vi "FPGAcode2_redo.vi"() -> ()   [LabVIEW 2015]
uses:
  IO_Cluster.ctl
  Limits_In.ctl
  <vilib>/Platform/TimedLoop/XDataNode/timing_clust.ctl
  <vilib>/Platform/TimedLoop/XDataNode/nitl_modes.ctl
  <vilib>/Platform/TimedLoop/XDataNode/wakeup.ctl
  <vilib>/rvi/Emulation/niFpgaGetClockAttributes.vi
  <vilib>/rvi/Emulation/niFpgaSctlEmulationGetInTimedLoop.vi
  <vilib>/rvi/Emulation/niFpgaEmulationReportErrorSimple.vi
  <vilib>/rvi/Emulation/niFpgaProcessEmulError.vi
  <vilib>/rvi/eio/common/nirviEmuTemplateMethod_errors.vi
  <vilib>/rvi/Emulation/niFpgaCriticalErrorInLSC.vi
  <vilib>/eio/EIONode/EIONode.xnode
  <vilib>/Platform/TimedLoop/XDataNode/XDataNode.xnode
  <vilib>/Platform/TimedLoop/XDataNode/XDNodeRunTimeDep.lvlib
panel:
  out "Delay":bool
  out "Plates":bool
  out "Offset Average":i16
  out "Boxcar Average":i16
  in  "Filter Thresholds":T1
  in  "Limits In":T2
  out "Detector 3 Correlations":T1
  out "Detector 1 Correlations":T1
  out "Del Armed":bool[](array[boolean])
  out "Armed":bool[](array[boolean])
  out "Delay Array":bool[](array[boolean])
  out "Plates Array":bool[](array[boolean])
  in  "Reset One Shot":bool
  in  "One Shot":bool
  in  "Mult1":fxp<+,16,7>
  out "IO Module\\AI 0":i16
  out "IO Module\\AI 1":i16
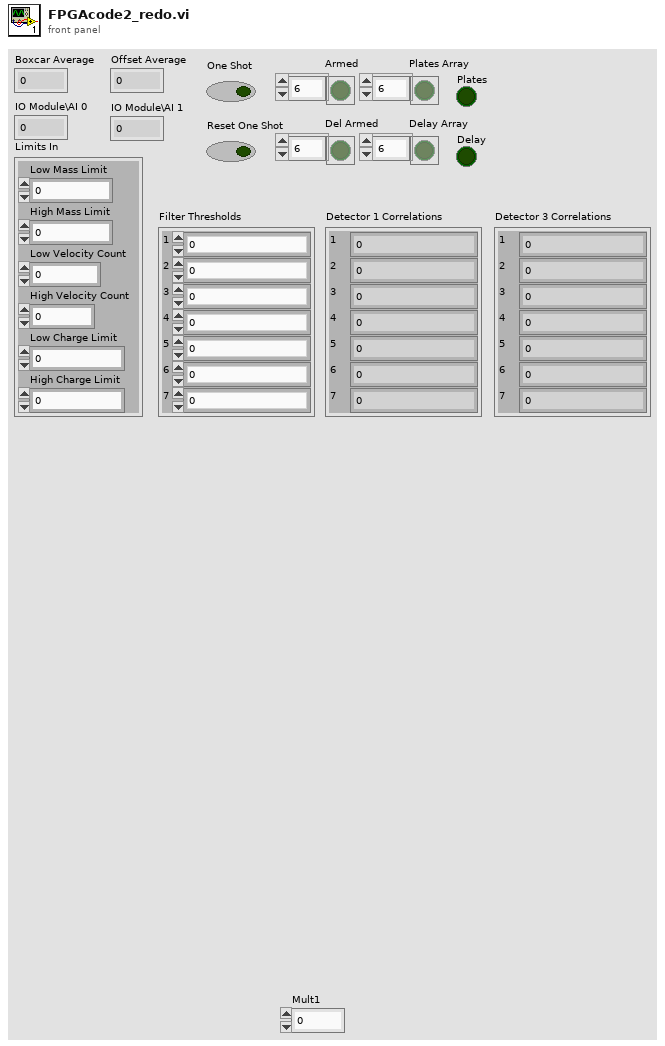
[diagram p1: front panel]
types:
  T1 = typedef "IO_Cluster.ctl" = cluster{"1":i16, "2":i16, "3":i16, "4":i16, "5":i16, "6":i16, "7":i16}
  T2 = typedef "Limits_In.ctl" = cluster{"Low Mass Limit":i64, "High Mass Limit":i64, "Low Velocity Count":i32, "High Velocity Count":i32, "Low Charge Limit":i16, "High Charge Limit":i16}
  T3 = typedef "XDNodeRunTimeDep.lvlib/timing_clust.ctl" = cluster{"Expected End [f-1]":u64, "Actual End [f-1]":u64, "Finished Late? [f-1]":bool, "Expected End [i-1]":u64, "Actual End [i-1]":u64, "Finished Late? [i-1]":bool, "Expected Start [i]":u64, "Actual Start [i]":u64, "Expected Start [f]":u64, "Actual Start [f]":u64, "Source Name":string, "Structure Name":string, "Period":i64, "Deadline":i64, "Offset":i64, "Start":i64, "Priority":i32, "Timeout":i32, "Mode":T4, "Wakeup Reason":T5, "Error":errorcluster, "Source Type":string, "Secondary Source Type":string, "Global End Time":u64, "Global Start Time":u64, "Frame Duration":u64, "Iteration Duration":u64, "Assigned CPU":i32, "I/O Scan Engine Mode":u32}
  T4 = typedef "XDNodeRunTimeDep.lvlib/nitl_modes.ctl" = enum32{"No Change", "Process missed periods, maintain original phase", "Discard missed periods, maintain original phase", "Process missed periods, ignore original phase", "Discard missed periods, ignore original phase"}
  T5 = typedef "XDNodeRunTimeDep.lvlib/wakeup.ctl" = enum32{"Normal", "Aborted", "Asynchronous wakeup", "Timing source error", "Timed loop error", "Timeout"}
  T6 = cluster{"High Charge Limit":i16, "Low Charge Limit":i16, "Time Out Limit":i32, "High Velocity Count":i32, "Low Velocity Count":i32, "Sampling Rate":fxp<+,30,25>, "High Mass Limit":i64, "Low Mass Limit":i64}
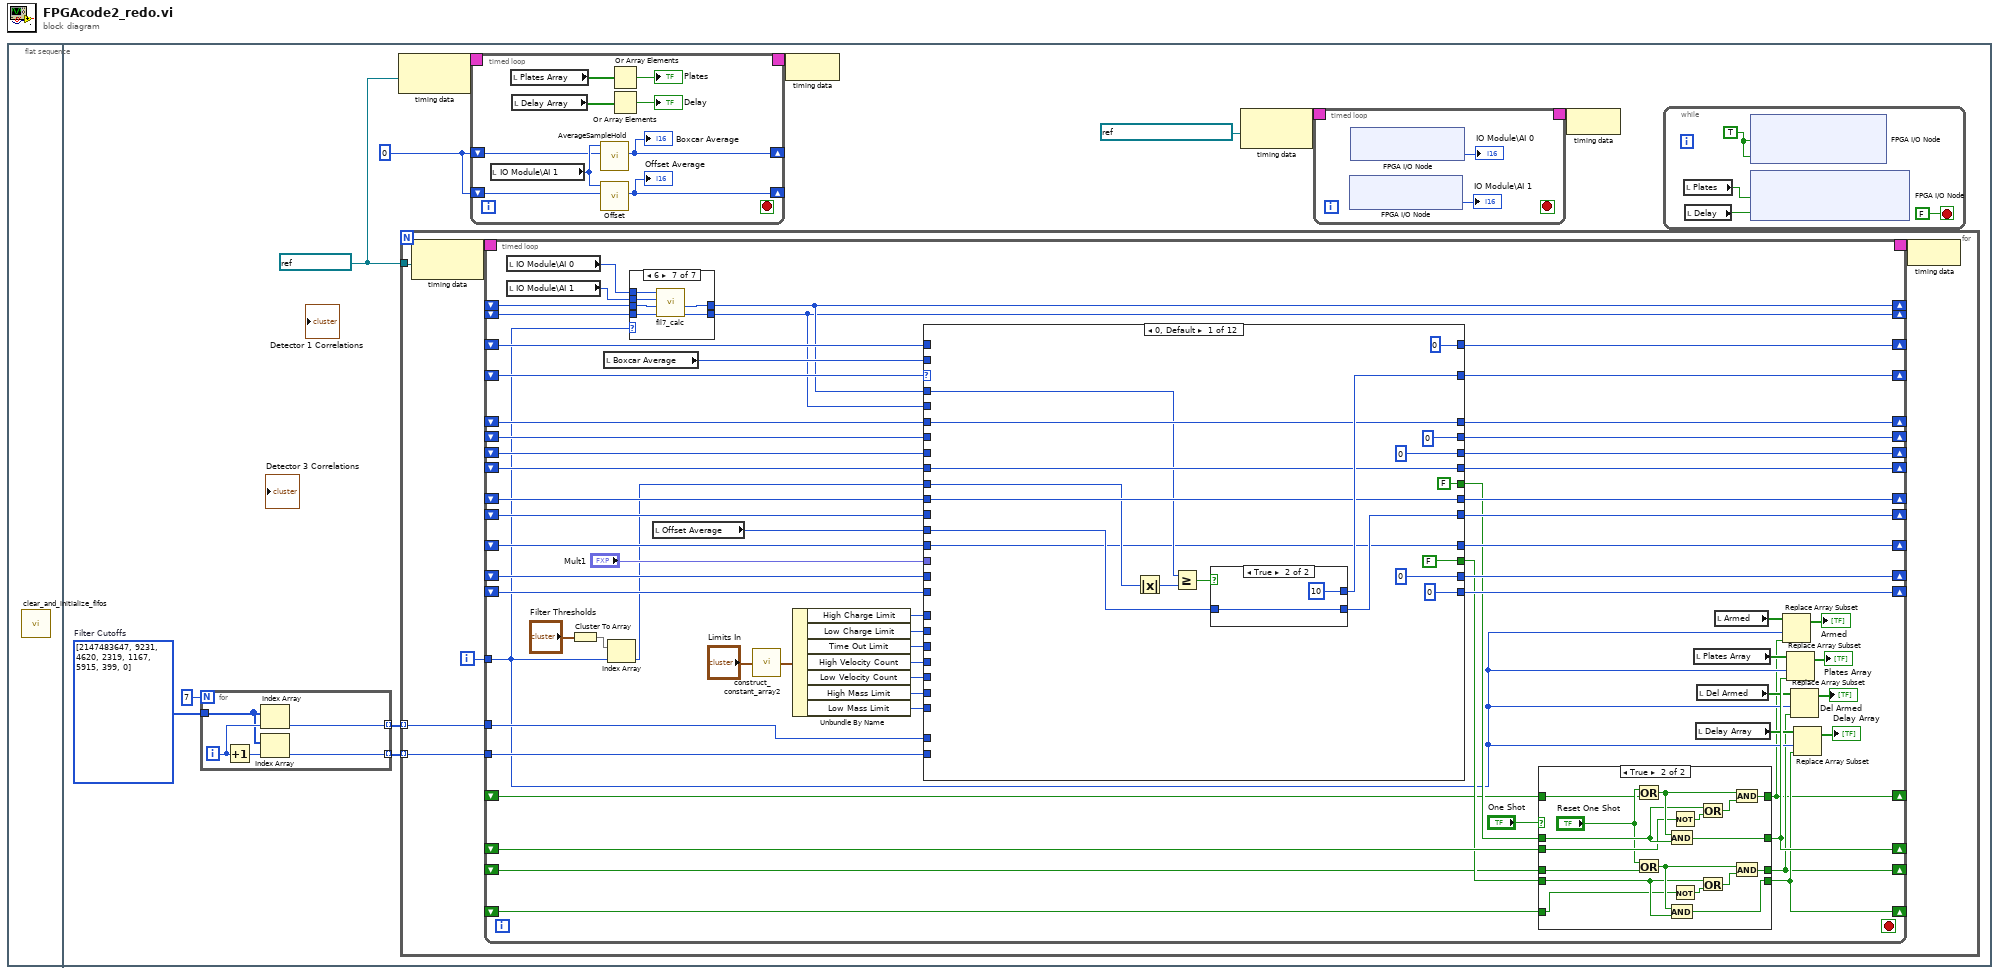
[diagram p0: block diagram]
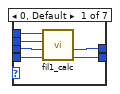
[diagram p2: hidden frame]
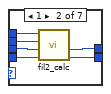
[diagram p3: hidden frame]
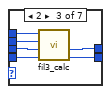
[diagram p4: hidden frame]
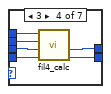
[diagram p5: hidden frame]
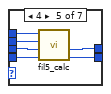
[diagram p6: hidden frame]
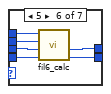
[diagram p7: hidden frame]
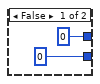
[diagram p8: hidden frame]
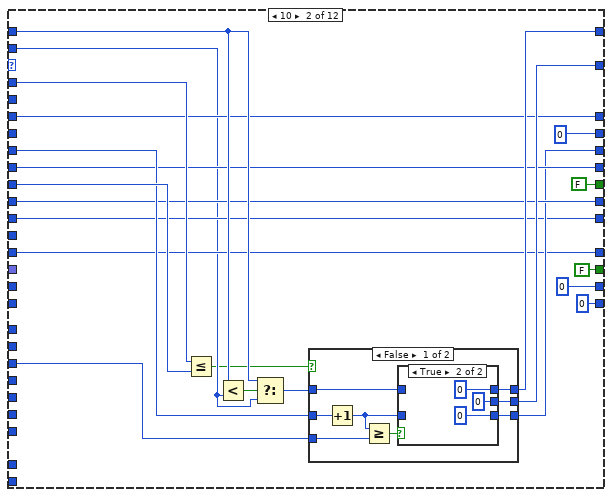
[diagram p9: hidden frame]
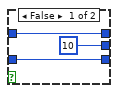
[diagram p10: hidden frame]
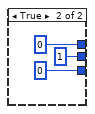
[diagram p11: hidden frame]
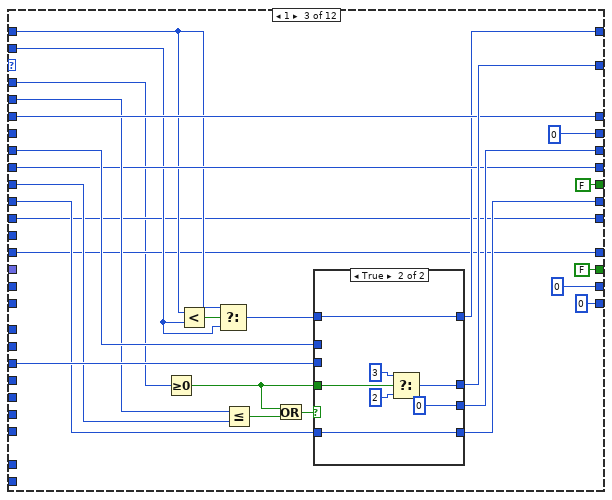
[diagram p12: hidden frame]
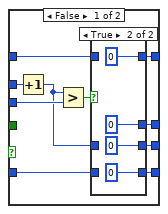
[diagram p13: hidden frame]
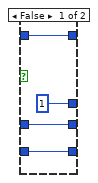
[diagram p14: hidden frame]
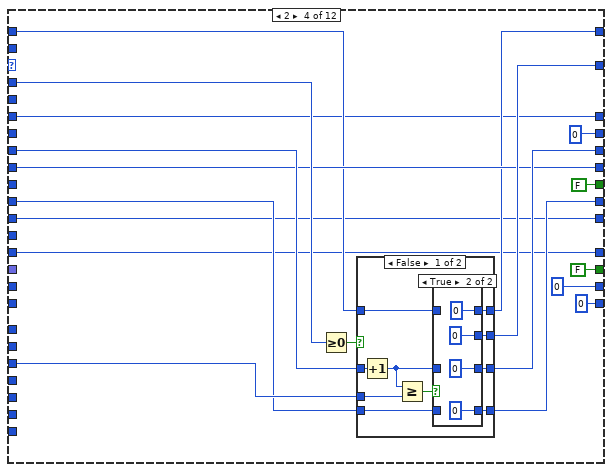
[diagram p15: hidden frame]
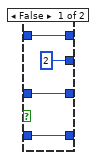
[diagram p16: hidden frame]
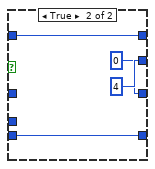
[diagram p17: hidden frame]
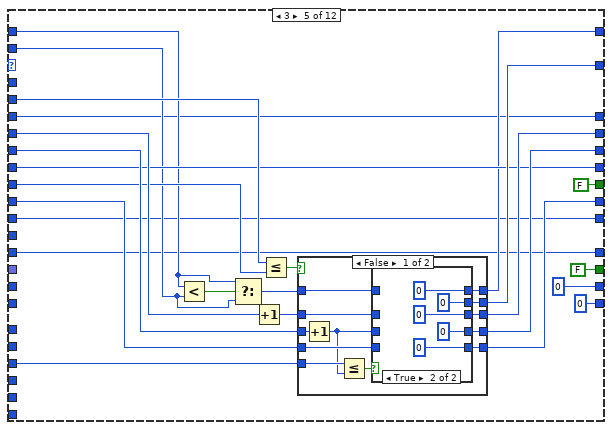
[diagram p18: hidden frame]
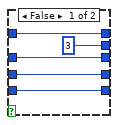
[diagram p19: hidden frame]
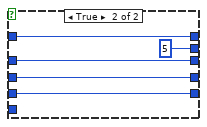
[diagram p20: hidden frame]
diagram:
  n1 = flat-sequence {
    frame #0 {
      n2 = call "clear_and_initialize_fifos.vi"() -> ()  [unwired: 1 in]
    }
    frame #1 {
      w1 = i16 0 ("Output New Average")
      w7 = i32[] [2147483647, 9231, 4620, 2319, 1167, 5915, 399, 0]  # Filter Cutoffs
      w2 = refnum<k21> "26.67MHz" ("Source Name")
      n3 = for {
        N: 7 -> [_]
        tunnel: w7 -> [w642]
        tunnel: [w641] -> w6 mode=indexing
        tunnel: [w640] -> w5 mode=indexing
        i -> [w644]
        n4 = Increment(x=w644) -> (x+1=w643:i32)
        n5 = Index Array(array=w642, index=w644) -> (element=w641:i32)
        n6 = Index Array(array=w642, index=w643) -> (element=w640:i32)
      }
      n7 = node-c288(w2) -> (w4:T3)
      n8 = for {
        tunnel: w2 -> [w30]
        tunnel: w6 -> [w29] mode=indexing
        tunnel: w5 -> [w28] mode=indexing
        i -> [w27]
        n9 = node-c288(w30) -> (w32:T3)
        n10 = timed-loop {
          timing: w32 -> [_]
          timing-out: [_] -> w31
          shift-right: [w67] -> _
          shift-left: _ -> [w66]
          shift-right: [w68] -> _
          shift-left: _ -> [w65]
          shift-right: [w69] -> _
          shift-left: _ -> [w64]
          shift-right: [w77] -> _
          shift-left: _ -> [w79]
          shift-right: [w76] -> _
          shift-left: _ -> [w80]
          shift-right: [w70] -> _
          shift-left: _ -> [w63]
          shift-right: [w71] -> _
          shift-left: _ -> [w62]
          shift-right: [w75] -> _
          shift-left: _ -> [w78]
          shift-right: [w72] -> _
          shift-left: _ -> [w61]
          shift-right: [w73] -> _
          shift-left: _ -> [w60]
          shift-right: [w74] -> _
          shift-left: _ -> [w59]
          shift-right: [w49] -> _
          shift-left: _ -> [w97]
          shift-right: [w42] -> _
          shift-left: _ -> [w47]
          shift-right: [w38] -> _
          shift-left: _ -> [w96]
          shift-right: [w39] -> _
          shift-left: _ -> [w95]
          tunnel: w29 -> [w94]
          tunnel: w28 -> [w93]
          tunnel: w27 -> [w37]
          shift-right: [w36] -> _
          shift-left: _ -> [w35]
          shift-right: [w34] -> _
          shift-left: _ -> [w33]
          stop <- _ stop-if-true
          n11 = local read "IO Module\\AI 0"() -> (w90:i16)
          n12 = local read "IO Module\\AI 1"() -> (w89:i16)
          n13 = Cluster To Array(cluster="Filter Thresholds") -> (array=w56:i16[])
          n14 = local read "Boxcar Average"() -> (w41:i16)
          n15 = Index Array(array=w56, index=w37) -> (element=w55:i16)
          n16 = case shown="6" w37 {
            tunnel: w96 -> [w103 w109 w115 w121 w127 w133 w139]
            tunnel: w95 -> [w102 w108 w114 w120 w126 w132 w138]
            tunnel: w90 -> [w101 w107 w113 w119 w125 w131 w137]
            tunnel: w89 -> [w100 w106 w112 w118 w124 w130 w136]
            tunnel: [w99 w105 w111 w117 w123 w129 w135] -> w39
            tunnel: [w98 w104 w110 w116 w122 w128 w134] -> w38
            frame 0, Default {
              n17 = call "fil1_calc.vi"("Detector 3 Correlation In"=w103, "Detector 1 Correlation In"=w102, "AI1"=w100, "AI0"=w101) -> ("Detector 3 Correlation Out"=w98:i16, "Detector 1 Correlation Out"=w99:i16)  [unwired: 4 in]
            }
            frame 1 {
              n18 = call "fil2_calc.vi"("Detector 3 Correlation In"=w109, "Detector 1 Correlation In"=w108, "AI1"=w106, "AI0"=w107) -> ("Detector 3 Correlation Out"=w104:i16, "Detector 1 Correlation Out"=w105:i16)  [unwired: 4 in]
            }
            frame 2 {
              n19 = call "fil3_calc.vi"("Detector 3 Correlation In"=w115, "Detector 1 Correlation In"=w114, "AI1"=w112, "AI0"=w113) -> ("Detector 3 Correlation Out"=w110:i16, "Detector 1 Correlation Out"=w111:i16)  [unwired: 4 in]
            }
            frame 3 {
              n20 = call "fil4_calc.vi"("Detector 3 Correlation In"=w121, "Detector 1 Correlation In"=w120, "AI1"=w118, "AI0"=w119) -> ("Detector 3 Correlation Out"=w116:i16, "Detector 1 Correlation Out"=w117:i16)  [unwired: 4 in]
            }
            frame 4 {
              n21 = call "fil5_calc.vi"("Detector 3 Correlation In"=w127, "Detector 1 Correlation In"=w126, "AI1"=w124, "AI0"=w125) -> ("Detector 3 Correlation Out"=w122:i16, "Detector 1 Correlation Out"=w123:i16)  [unwired: 4 in]
            }
            frame 5 {
              n22 = call "fil6_calc.vi"("Detector 3 Correlation In"=w133, "Detector 1 Correlation In"=w132, "AI1"=w130, "AI0"=w131) -> ("Detector 3 Correlation Out"=w128:i16, "Detector 1 Correlation Out"=w129:i16)  [unwired: 4 in]
            }
            frame 6 {
              n23 = call "fil7_calc.vi"("Detector 3 Correlation In"=w139, "Detector 1 Correlation In"=w138, "AI1"=w136, "AI0"=w137) -> ("Detector 3 Correlation Out"=w134:i16, "Detector 1 Correlation Out"=w135:i16)  [unwired: 4 in]
            }
          }
          n24 = local read "Offset Average"() -> (w40:i16)
          n25 = call "construct_constant_array2.vi"("Limits In"="Limits In") -> ("Limits Out"=w81:T6)
          n26 = Unbundle By Name(w81) -> ("High Charge Limit"=w82:i16, "Low Charge Limit"=w83:i16, "Time Out Limit"=w84:i32, "High Velocity Count"=w85:i32, "Low Velocity Count"=w86:i32, "High Mass Limit"=w87:i64, "Low Mass Limit"=w88:i64)
          n27 = case shown="0, Default" w65 {
            tunnel: w39 -> [w151 w181 w202 w266 _ _ _ _ _ _ _ _]
            tunnel: w38 -> [_ _ w219 _ w310 w358 w405 _ _ _ _ _]
            tunnel: w55 -> [w149 w180 w218 _ w309 _ _ _ _ _ _ _]
            tunnel: w63 -> [_ _ _ _ w312 w365 w414 w456 w513 w542 w572 _]
            tunnel: [0 0 0 0 w317 w364 w407 w441 w512 w540 w570 0] -> w70
            tunnel: [w157 w179 w226 w270 w316 w361 w410 w461 w511 w541 w571 w596] -> w68
            tunnel: w64 -> [w155 w174 w220 w258 w298 w350 w406 w462 w487 w526 w568 w587]
            tunnel: w84 -> [_ w177 w225 w269 w314 w359 w411 _ _ _ _ _]
            tunnel: w62 -> [_ w178 w224 w268 w315 w360 w413 _ _ _ _ _]
            tunnel: [u32 0 w169 w223 w267 w313 w362 w409 u32 0 u32 0 ("Timeout Count in") u32 0 ("Timeout Count in") u32 0 u32 0 ("Timeout Count in")] -> w71
            tunnel: w86 -> [_ _ _ _ _ _ _ _ w510 _ _ _]
            tunnel: w85 -> [_ _ _ _ _ _ _ _ w509 _ _ _]
            tunnel: [w155 w174 w220 w258 w298 w350 w406 w463 w487 w526 w568 w587] -> w69
            tunnel: w83 -> [_ _ _ _ _ _ _ _ w508 _ _ _]
            tunnel: w82 -> [_ _ _ _ _ _ _ _ w507 _ _ _]
            tunnel: w60 -> [w154 w171 w217 w265 w308 w353 w404 w459 w506 w538 w566 _]
            tunnel: [w154 w171 w216 w264 w307 w357 w403 w460 w505 w538 w567 0 ("Noise Level")] -> w73
            tunnel: w61 -> [w153 w172 w215 w263 w306 w356 w402 w458 w488 w534 w563 w589]
            tunnel: [w153 w172 w215 w263 w306 w356 w402 w458 w488 w535 w563 w589] -> w72
            tunnel: [0 ("Old Average In") w175 w214 w262 w305 w355 w401 w457 w501 w531 0 ("Old Average In") 0 ("Old Average In")] -> w67
            tunnel: w94 -> [_ _ _ _ _ _ _ w443 _ _ _ _]
            tunnel: w93 -> [_ _ _ _ _ _ _ w442 _ _ _ _]
            tunnel: [FALSE FALSE ("Data") FALSE FALSE FALSE FALSE FALSE FALSE FALSE ("Data") w525 w557 FALSE ("Data")] -> w54
            tunnel: w66 -> [_ w182 w211 w260 w302 w352 w399 w453 w501 w531 _ _]
            tunnel: w41 -> [_ w163 w210 _ w301 _ _ _ _ _ _ _]
            tunnel: w59 -> [_ w168 w208 w259 w299 w351 w398 w452 w502 w530 _ _]
            tunnel: w40 -> [w146 _ _ _ _ _ _ _ _ _ _ _]
            tunnel: [w147 w168 w208 w259 w299 w351 w398 w452 w502 w530 0 ("Offset") 0 ("Offset")] -> w74
            tunnel: [w145 w167 w207 w257 w297 w349 w397 w451 w489 w536 w561 w594] -> w75
            tunnel: w78 -> [w145 w167 w207 w257 w297 w349 w397 w451 w489 w537 w561 w594]
            tunnel: w87 -> [_ _ _ _ _ _ _ _ w500 _ _ _]
            tunnel: w88 -> [_ _ _ _ _ _ _ _ w499 _ _ _]
            tunnel: w80 -> [_ _ _ _ _ _ _ _ w495 w529 w560 w585]
            tunnel: [0 0 0 0 0 0 0 w447 w494 w527 w555 w582] -> w77
            tunnel: [FALSE FALSE FALSE FALSE FALSE FALSE FALSE FALSE FALSE w524 w556 w586] -> w48
            tunnel: [u16 0 u16 0 u16 0 u16 0 u16 0 u16 0 u16 0 u16 0 u16 0 u16 0 w559 w595] -> w76
            tunnel: w79 -> [_ _ _ _ _ _ _ _ _ _ _ w583]
            tunnel: "Mult1" -> [_ _ _ _ _ _ _ w446 _ _ _ _]
            frame 0, Default {
              n28 = Absolute Value(x=w149) -> (abs(x)=w148:i16)
              n29 = Greater Or Equal?(x=w151, y=w148) -> (x >= y?=w140:bool)
              n30 = case shown="True" w140 {
                tunnel: [u8 0 u8 10] -> w157
                tunnel: [0 w160] -> w147
                tunnel: w146 -> [_ w160]
                frame False {
                }
                frame True {
                }
              }
            }
            frame 10 {
              n31 = Less Or Equal?(x=w181, y=w180) -> (x <= y?=w162:bool)
              n32 = Less?(x=w182, y=w163) -> (x < y?=w183:bool)
              n33 = Select(t=w182, s=w183, f=w163) -> (s? t:f=w176:i32)
              n34 = case shown="False" w162 {
                tunnel: [w189 u8 1] -> w179
                tunnel: w178 -> [w186 _]
                tunnel: w177 -> [w191 _]
                tunnel: w176 -> [w188 _]
                tunnel: [w187 0 ("New Average")] -> w175
                tunnel: [w184 0] -> w169
                frame False {
                  n35 = Increment(x=w186) -> (x+1=w185:u32)
                  n36 = Greater Or Equal?(x=w185, y=w191) -> (x >= y?=w190:bool)
                  n37 = case shown="True" w190 {
                    tunnel: [u8 10 u8 0] -> w189
                    tunnel: w188 -> [w194 _]
                    tunnel: [w194 0 ("New Average")] -> w187
                    tunnel: w185 -> [w192 _]
                    tunnel: [w192 0] -> w184
                    frame False {
                    }
                    frame True {
                    }
                  }
                }
                frame True {
                }
              }
            }
            frame 1 {
              n38 = Greater Or Equal To 0?(x=w202) -> (x >= 0?=w222:bool)
              n39 = Less?(x=w211, y=w210) -> (x < y?=w212:bool)
              n40 = Select(t=w211, s=w212, f=w210) -> (s? t:f=w209:i32)
              n41 = Less Or Equal?(x=w219, y=w218) -> (x <= y?=w221:bool)
              n42 = Or(x=w222, y=w221) -> (x .or. y?=w201:bool)
              n43 = case shown="True" w201 {
                tunnel: [w234 w246] -> w226
                tunnel: w225 -> [w236 _]
                tunnel: w224 -> [w233 _]
                tunnel: [w232 u32 0] -> w223
                tunnel: w222 -> [_ w245]
                tunnel: w217 -> [w231 w250]
                tunnel: [w230 w250] -> w216
                tunnel: [w229 w251] -> w214
                tunnel: w209 -> [w227 w251]
                frame False {
                  n44 = Increment(x=w233) -> (x+1=w228:u32)
                  n45 = Greater?(x=w228, y=w236) -> (0:w235:bool)
                  n46 = case shown="True" w235 {
                    tunnel: [u8 1 u8 0 ("Old Average In")] -> w234
                    tunnel: w228 -> [w239 _]
                    tunnel: [w239 u32 0 ("Old Average In")] -> w232
                    tunnel: w231 -> [w238 _]
                    tunnel: [w238 0 ("Old Average In")] -> w230
                    tunnel: [w237 0 ("Old Average In")] -> w229
                    tunnel: w227 -> [w237 _]
                    frame False {
                    }
                    frame True {
                    }
                  }
                }
                frame True {
                  n47 = Select(t=u8 3, s=w245, f=u8 2) -> (s? t:f=w246:u8)
                }
              }
            }
            frame 2 {
              n48 = Greater Or Equal To 0?(x=w266) -> (x >= 0?=w252:bool)
              n49 = case shown="False" w252 {
                tunnel: [w279 u8 4] -> w270
                tunnel: w269 -> [w278 _]
                tunnel: w268 -> [w276 _]
                tunnel: [w277 u32 0] -> w267
                tunnel: w265 -> [w275 w290]
                tunnel: [w274 w290] -> w264
                tunnel: [w273 w289] -> w262
                tunnel: w260 -> [w272 w289]
                frame False {
                  n50 = Increment(x=w276) -> (x+1=w271:u32)
                  n51 = Greater Or Equal?(x=w271, y=w278) -> (x >= y?=w280:bool)
                  n52 = case shown="True" w280 {
                    tunnel: [u8 2 u8 0] -> w279
                    tunnel: w271 -> [w284 _]
                    tunnel: [w284 u32 0] -> w277
                    tunnel: w275 -> [w282 _]
                    tunnel: [w282 0 ("High Correlation In")] -> w274
                    tunnel: [w281 0 ("Old Average In")] -> w273
                    tunnel: w272 -> [w281 _]
                    frame False {
                    }
                    frame True {
                    }
                  }
                }
                frame True {
                }
              }
            }
            frame 3 {
              n53 = Less?(x=w302, y=w301) -> (x < y?=w303:bool)
              n54 = Select(t=w302, s=w303, f=w301) -> (s? t:f=w300:i32)
              n55 = Increment(x=w312) -> (x+1=w311:i32)
              n56 = Less Or Equal?(x=w310, y=w309) -> (x <= y?=w293:bool)
              n57 = case shown="False" w293 {
                tunnel: w311 -> [w325 w344]
                tunnel: [w324 w344] -> w317
                tunnel: [w327 u8 5] -> w316
                tunnel: w315 -> [w323 w340]
                tunnel: w314 -> [w329 _]
                tunnel: [w326 w340] -> w313
                tunnel: w308 -> [w322 w342]
                tunnel: [w321 w342] -> w307
                tunnel: [w320 w341] -> w305
                tunnel: w300 -> [w319 w341]
                frame False {
                  n58 = Increment(x=w323) -> (x+1=w318:u32)
                  n59 = Less Or Equal?(x=w329, y=w318) -> (x <= y?=w328:bool)
                  n60 = case shown="True" w328 {
                    tunnel: [u8 3 u8 0] -> w327
                    tunnel: w318 -> [w333 _]
                    tunnel: [w333 u32 0] -> w326
                    tunnel: w325 -> [w332 _]
                    tunnel: [w332 0] -> w324
                    tunnel: w322 -> [w331 _]
                    tunnel: [w331 0 ("High Correlation In")] -> w321
                    tunnel: [w330 0 ("Old Average In")] -> w320
                    tunnel: w319 -> [w330 _]
                    frame False {
                    }
                    frame True {
                    }
                  }
                }
                frame True {
                }
              }
            }
            frame 4 {
              n61 = Greater Or Equal To 0?(x=w358) -> (x >= 0?=w345:bool)
              n62 = Increment(x=w365) -> (x+1=w363:i32)
              n63 = case shown="True" w345 {
                tunnel: [w370 w392] -> w364
                tunnel: w363 -> [w371 w392]
                tunnel: [w373 u32 0] -> w362
                tunnel: [w375 u8 6] -> w361
                tunnel: w360 -> [w377 _]
                tunnel: w359 -> [w372 _]
                tunnel: w353 -> [w369 w389]
                tunnel: [w368 w389] -> w357
                tunnel: [w367 w388] -> w355
                tunnel: w352 -> [w366 w388]
                frame False {
                  n64 = Increment(x=w377) -> (x+1=w374:u32)
                  n65 = Greater Or Equal?(x=w374, y=w372) -> (x >= y?=w376:bool)
                  n66 = case shown="True" w376 {
                    tunnel: [u8 4 u8 0] -> w375
                    tunnel: w374 -> [w381 _]
                    tunnel: [w381 u32 0] -> w373
                    tunnel: w371 -> [w380 _]
                    tunnel: [w380 0] -> w370
                    tunnel: w369 -> [w379 _]
                    tunnel: [w379 0 ("High Correlation In")] -> w368
                    tunnel: [w378 0 ("Old Average In")] -> w367
                    tunnel: w366 -> [w378 _]
                    frame False {
                    }
                    frame True {
                    }
                  }
                }
                frame True {
                }
              }
            }
            frame 5 {
              n67 = Increment(x=w413) -> (x+1=w412:u32)
              n68 = Greater Or Equal To 0?(x=w405) -> (x >= 0?=w393:bool)
              n69 = Increment(x=w414) -> (x+1=w408:i32)
              n70 = case shown="False" w393 {
                tunnel: w412 -> [w421 _]
                tunnel: w411 -> [w425 _]
                tunnel: [w423 u8 6] -> w410
                tunnel: [w422 u32 0] -> w409
                tunnel: w408 -> [w420 w438]
                tunnel: [w419 w438] -> w407
                tunnel: w404 -> [w417 w437]
                tunnel: [w418 w437] -> w403
                tunnel: [w416 w436] -> w401
                tunnel: w399 -> [w415 w436]
                frame False {
                  n71 = Greater Or Equal?(x=w421, y=w425) -> (x >= y?=w424:bool)
                  n72 = case shown="True" w424 {
                    tunnel: [u8 5 u8 0] -> w423
                    tunnel: [w429 u32 0] -> w422
                    tunnel: w421 -> [w429 _]
                    tunnel: w420 -> [w428 _]
                    tunnel: [w428 0] -> w419
                    tunnel: [w427 0 ("High Correlation In")] -> w418
                    tunnel: w417 -> [w427 _]
                    tunnel: [w426 0 ("Old Average In")] -> w416
                    tunnel: w415 -> [w426 _]
                    frame False {
                    }
                    frame True {
                    }
                  }
                }
                frame True {
                }
              }
            }
            frame 6 {
              n73 = Less?(x=w456, y=w443) -> (x < y?=w445:bool)
              n74 = Greater Or Equal?(x=w456, y=w442) -> (x >= y?=w444:bool)
              n75 = And(x=w445, y=w444) -> (x .and. y?=w455:bool)
              n76 = case shown="True" w455 {
                tunnel: [0 w473] -> w441
                tunnel: w456 -> [_ w472]
                tunnel: [w469 w472] -> w463
                tunnel: w462 -> [w469 _]
                tunnel: [u8 0 u8 7] -> w461
                tunnel: [0 ("High Correlation In") w477] -> w460
                tunnel: w459 -> [_ w477]
                tunnel: [0 ("Old Average In") w476] -> w457
                tunnel: w453 -> [_ w476]
                frame False {
                }
                frame True {
                  n77 = Multiply(x=w472, y=fxp<+,6,1> 1.40625) -> (x*y=w471:fxp<+/-,38,33>)
                  n78 = To Long Integer(number=w471) -> (32bit integer=w470:i32)
                  n79 = Subtract(x=w470, y=19) -> (x-y=w473:i32)
                }
              }
              n80 = Multiply(x=w441, y=w446) -> (x*y=w449:fxp<+/-,48,39>)
              n81 = To Long Integer(number=w449) -> (32bit integer=w447:i32)
            }
            frame 7 {
              n82 = Square(x=w487) -> (x^2=w483:i32)
              n83 = Subtract(x=w502, y=w501) -> (x-y=w504:i32)
              n84 = To Quad Integer(1:w483) -> (0:w496:i64)
              n85 = Absolute Value(x=w504) -> (abs(x)=w482:i32)
              n86 = To Quad Integer(1:w482) -> (0:w497:i64)
              n87 = Greater Or Equal?(x=w507, y=w482) -> (x >= y?=w486:bool)
              n88 = Less Or Equal?(x=w508, y=w482) -> (x <= y?=w485:bool)
              n89 = Multiply(x=w497, y=w496) -> (x*y=w498:i64)
              n90 = Greater Or Equal?(x=w487, y=w509) -> (x >= y?=w484:bool)
              n91 = Less Or Equal?(x=w487, y=w510) -> (x <= y?=w481:bool)
              n92 = Less Or Equal?(x=w498, y=w500) -> (x <= y?=w479:bool)
              n93 = Greater Or Equal?(x=w498, y=w499) -> (x >= y?=w480:bool)
              n94 = Compound Arithmetic op=AND(w486, w485, w484, w481, w479, w480) -> (w503:bool)
              n95 = case shown="True" w503 {
                tunnel: w513 -> [_ w523]
                tunnel: [0 w521] -> w512
                tunnel: [u8 0 u8 8] -> w511
                tunnel: w506 -> [_ w522]
                tunnel: [0 ("High Correlation In") w522] -> w505
                tunnel: w495 -> [_ w519]
                tunnel: [0 w518] -> w494
                frame False {
                }
                frame True {
                  n96 = Decrement(x=w523) -> (x-1=w521:i32)
                  n97 = Decrement(x=w519) -> (x-1=w518:i32)
                }
              }
            }
            frame 8 {
              n98 = Decrement(x=w542) -> (x-1=w543:i32)
              n99 = Subtract(x=w530, y=w531) -> (x-y=w533:i32)
              n100 = Less Or Equal To 0?(x=w543) -> (x <= 0?=w525:bool)
              n101 = Absolute Value(x=w533) -> (abs(x)=w532:i32)
              n102 = case shown="True" w525 {
                tunnel: [u8 8 u8 9] -> w541
                tunnel: [w547 w553] -> w540
                tunnel: w526 -> [_ w551]
                tunnel: w543 -> [w547 _]
                tunnel: w537 -> [w545 _]
                tunnel: [w545 w551] -> w536
                tunnel: [w544 w550] -> w535
                tunnel: w534 -> [w544 _]
                tunnel: w532 -> [_ w550]
                frame False {
                }
                frame True {
                  n103 = To Fixed-Point(number=w551) -> (fixed-point=w548:fxp<+/-,32,32>)  [unwired: 1 in]
                  n104 = Multiply(x=fxp<+,2,1> 1.5, y=w548) -> (x*y=w554:fxp<+/-,34,33>)
                  n105 = To Long Integer(number=w554) -> (32bit integer=w553:i32)
                }
              }
              n106 = Decrement(x=w529) -> (x-1=w527:i32)
              n107 = Less Or Equal To 0?(x=w527) -> (x <= 0?=w524:bool)
            }
            frame 9 {
              n108 = Decrement(x=w572) -> (x-1=w569:i32)
              n109 = Less Or Equal To 0?(x=w569) -> (x <= 0?=w558:bool)
              n110 = case shown="True" w558 {
                tunnel: [w575 0] -> w570
                tunnel: [u8 9 u8 12] -> w571
                tunnel: w569 -> [w575 _]
                tunnel: w566 -> [w574 _]
                tunnel: [w574 0 ("Noise Level")] -> w567
                tunnel: [u16 0 u16 550] -> w559
                frame False {
                }
                frame True {
                }
              }
              n111 = Decrement(x=w560) -> (x-1=w555:i32)
              n112 = Not(x=w558) -> (.not. x?=w557:bool)
              n113 = Less Or Equal To 0?(x=w555) -> (x <= 0?=w556:bool)
            }
            frame 12 {
              n114 = Decrement(x=w585) -> (x-1=w581:i32)
              n115 = Less Or Equal To 0?(x=w581) -> (x <= 0?=w584:bool)
              n116 = case shown="True" w584 {
                tunnel: [FALSE w602] -> w586
                tunnel: [u8 12 w607] -> w596
                tunnel: w583 -> [w600 w608]
                tunnel: [w600 w606] -> w595
                tunnel: [w598 0] -> w582
                tunnel: w581 -> [w598 _]
                frame False {
                }
                frame True {
                  n117 = Decrement(x=w608) -> (x-1=w605:i32)
                  n118 = Less Or Equal To 0?(x=w605) -> (x <= 0?=w603:bool)
                  n119 = case shown="False" w603 {
                    tunnel: [u8 12 u8 0] -> w607
                    tunnel: [w609 u16 0] -> w606
                    tunnel: w605 -> [w609 _]
                    frame False {
                    }
                    frame True {
                    }
                  }
                  n120 = Not(x=w603) -> (.not. x?=w602:bool)
                }
              }
            }
          }
          n121 = case shown="True" "One Shot" {
            tunnel: [w616 w631] -> w49
            tunnel: w54 -> [w616 w628]
            tunnel: [FALSE w633] -> w34
            tunnel: w97 -> [_ w627]
            tunnel: [FALSE w623] -> w36
            tunnel: [w613 w622] -> w42
            tunnel: w48 -> [w613 w621]
            tunnel: w47 -> [_ w620]
            tunnel: w35 -> [_ w619]
            tunnel: w33 -> [_ w617]
            frame False {
            }
            frame True {
              n122 = Or(x="Reset One Shot", y=w617) -> (x .or. y?=w632:bool)
              n123 = Or(x="Reset One Shot", y=w619) -> (x .or. y?=w624:bool)
              n124 = And(x=w632, y=w628) -> (x .and. y?=w631:bool)
              n125 = And(x=w624, y=w621) -> (x .and. y?=w622:bool)
              n126 = Not(x=w627) -> (.not. x?=w629:bool)
              n127 = Not(x=w620) -> (.not. x?=w626:bool)
              n128 = Or(x=w628, y=w629) -> (x .or. y?=w630:bool)
              n129 = Or(x=w621, y=w626) -> (x .or. y?=w625:bool)
              n130 = And(x=w632, y=w630) -> (x .and. y?=w633:bool)
              n131 = And(x=w624, y=w625) -> (x .and. y?=w623:bool)
            }
          }
          n132 = local read "Plates Array"() -> (w51:bool[])
          n133 = local read "Delay Array"() -> (w46:bool[])
          n134 = local read "Del Armed"() -> (w45:bool[])
          n135 = local read "Armed"() -> (w53:bool[])
          n136 = Replace Array Subset(array=w53, new element=w34, index=w37) -> (→"Armed":bool[])
          n137 = Replace Array Subset(array=w51, new element=w49, index=w37) -> (→"Plates Array":bool[])
          n138 = Replace Array Subset(array=w45, new element=w36, index=w37) -> (→"Del Armed":bool[])
          n139 = Replace Array Subset(array=w46, new element=w42, index=w37) -> (→"Delay Array":bool[])
        }
        n140 = node-c288(w31) -> ()
      }
      n141 = timed-loop {
        timing: w4 -> [_]
        timing-out: [_] -> w3
        shift-right: [w16] -> _
        shift-left: w1 -> [w19]
        shift-right: [w18] -> _
        shift-left: w1 -> [w17]
        stop <- _ stop-if-true
        n142 = local read "IO Module\\AI 1"() -> (w20:i16)
        n143 = local read "Plates Array"() -> (w15:bool[])
        n144 = local read "Delay Array"() -> (w14:bool[])
        n145 = call "AverageSampleHold.vi"("Previous Average"=w17, "Input Value"=w20) -> ("Output New Average"=w18:i16)  [unwired: 9 in]
        "Boxcar Average" <- w18
        n146 = call "Offset.vi"("Previous Average"=w19, "Input Value"=w20) -> ("Output New Average"=w16:i16)  [unwired: 9 in]
        "Offset Average" <- w16
        n147 = Or Array Elements(Boolean array=w15) -> (logical OR=→"Plates":bool)
        n148 = Or Array Elements(Boolean array=w14) -> (logical OR=→"Delay":bool)
      }
      n149 = node-c288(w3) -> ()
      n150 = node-c288(refnum<k21> "IO Module\\Data Clock" ("Source Name")) -> (w11:T3)
      n151 = timed-loop {
        timing: w11 -> [_]
        timing-out: [_] -> w10
        stop <- _ stop-if-true
        n152 = xnode "FPGA I/O Node"() -> ("IO Module\\AI 1"=→"IO Module\\AI 1":i16)  [unwired: 1 in, 1 out]
        n153 = xnode "FPGA I/O Node"() -> ("IO Module\\AI 0"=→"IO Module\\AI 0":i16)  [unwired: 1 in, 1 out]
      }
      n154 = node-c288(w10) -> ()
      n155 = while {
        stop <- FALSE stop-if-true
        w656 = TRUE ("IO Module\\PFI Enable")
        n156 = local read "Plates"() -> (w654:bool)
        n157 = local read "Delay"() -> (w653:bool)
        n158 = xnode "FPGA I/O Node"("IO Module\\PFI 0 WE"=w656, "IO Module\\PFI 1 WE"=w656) -> ()  [unwired: 2 in, 2 out]
        n159 = xnode "FPGA I/O Node"("IO Module\\PFI 0 Wr Data"=w654, "IO Module\\PFI 1 Wr Data"=w653) -> ()  [unwired: 2 in, 2 out]
      }
    }
  }
